vi "Plot Field Calibration.vi"(9 "Step":dbl, 10 "Max Field":dbl, 11 "Field Calibration":T1 {"x locations" format="%.4g"; "coefficients" format="%.4g"}) -> (1 "Field Calibration Plot":cluster{dbl[], dbl[]}(graph))   [LabVIEW 2012, in "Varian.lvlib"]
doc: "Creates a plot of the given Field Calibration from the provided extrapolated function."
uses:
  Varian.lvlib
  <vilib>/gmath/interp.llb/in_piecewise interp poly control.ctl
  <vilib>/gmath/NI_Gmath.lvlib
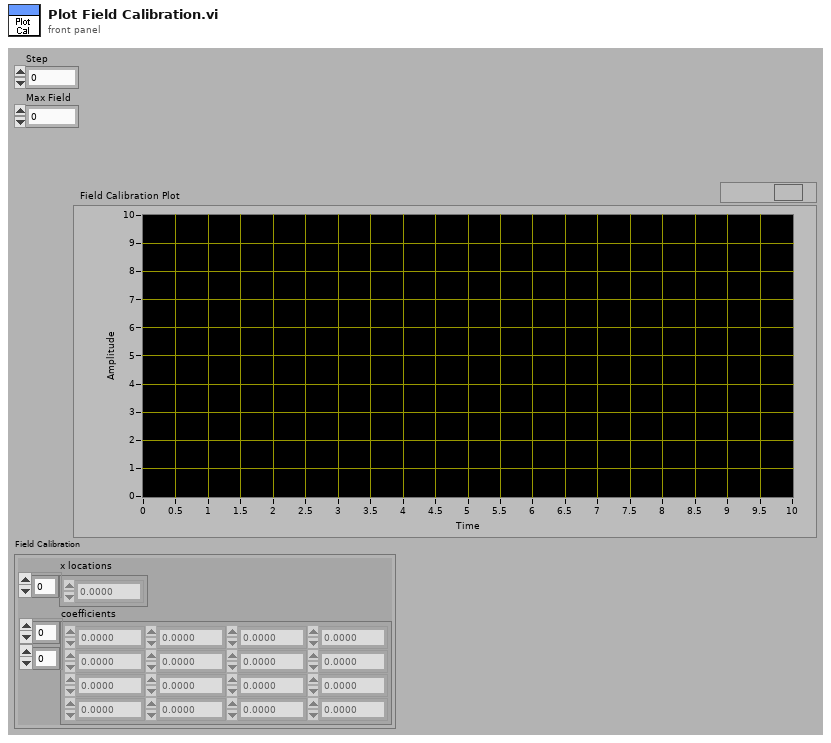
[diagram p1: front panel]
types:
  T1 = typedef "NI_Gmath.lvlib/in_piecewise interp poly control.ctl" = cluster{"x locations":dbl[], "coefficients":dbl[][]}
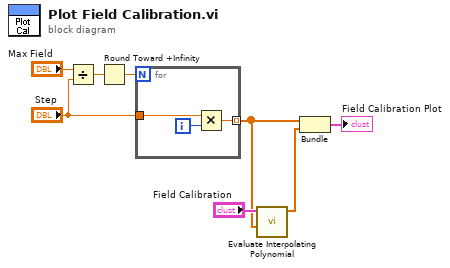
[diagram p0: block diagram]
diagram:
  n1 = Divide(x="Max Field", y="Step") -> (x/y=w5:dbl)
  n2 = Round Toward +Infinity(x=w5) -> (ceil(x): smallest int >= x=w6:dbl)
  n3 = for {
    N: w6 -> [_]
    tunnel: [w9] -> w3 mode=indexing
    tunnel: "Step" -> [w10]
    i -> [w11]
    n4 = Multiply(x=w10, y=w11) -> (x*y=w9:dbl)
  }
  n5 = call <vilib>:"Evaluate Interpolating Polynomial.vi"("xi"=w3, "piecewise polynomial"="Field Calibration") -> ("yi"=w2:dbl[])  [unwired: 8 in, 1 out]
  n6 = Bundle(w3, "yi"=w2) -> (→"Field Calibration Plot":cluster{dbl[], "yi":dbl[]})  [unwired: 1 in]
